vi "Slide Change Display Format.vi"(8 "Error In":errorcluster, 11 "Slide Refnum":refnum<vi>) -> (0 "Error Out":errorcluster)   [LabVIEW 2021, in "GUI.lvlib"]
uses:
  GUI.lvlib
panel:
  # "see the License on the block diagram (Ctrl+E or Window:Show Block Diagram)"
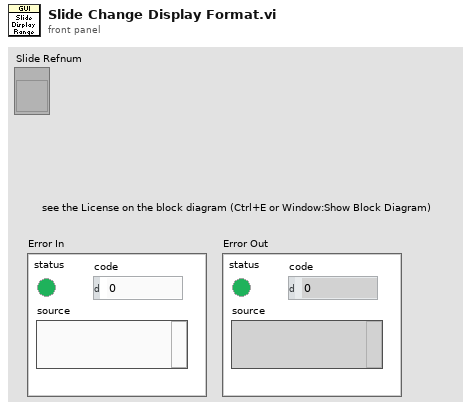
[diagram p1: front panel]
types:
  T1 = typedef "LVFormatAndPrecisionTypeDef.ctl" = cluster{"Format":u8, "Precision":u8}
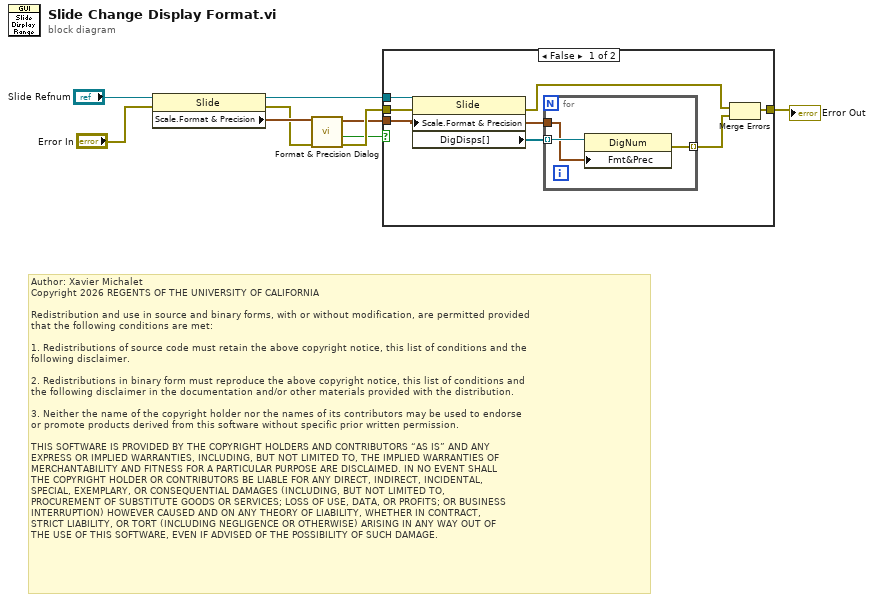
[diagram p0: block diagram]
diagram:
  # "Author: Xavier Michalet\nCopyright 2026 REGENTS OF THE UNIVERSITY OF CALIFORNIA\n\nRedistribution and use in source and binary forms, with or without modification, are permitted provided\nthat the following conditions are met:\n\n1. Redistributions of source code must retain the above copyright notice, this list of conditions and the\nfollowing disclaimer.\n\n2. Redistributions in binary form must reproduce the above copyright notice, this list of conditions and\nthe following disclaimer in the documentation and/or other materials provided with the distribution.\n\n3. Neither the name of the copyright holder nor the names of its contributors may be used to endorse \nor promote products derived from this software without specific prior written permission.\n\nTHIS SOFTWARE IS PROVIDED BY THE COPYRIGHT HOLDERS AND CONTRIBUTORS “AS IS” AND ANY \nEXPRESS OR IMPLIED WARRANTIES, INCLUDING, BUT NOT LIMITED TO, THE IMPLIED WARRANTIES OF\nMERCHANTABILITY AND FITNESS FOR A PARTICULAR PURPOSE ARE DISCLAIMED. IN NO EVENT SHALL\nTHE COPYRIGHT HOLDER OR CONTRIBUTORS BE LIABLE FOR ANY DIRECT, INDIRECT, INCIDENTAL, \nSPECIAL, EXEMPLARY, OR CONSEQUENTIAL DAMAGES (INCLUDING, BUT NOT LIMITED TO, \nPROCUREMENT OF SUBSTITUTE GOODS OR SERVICES; LOSS OF USE, DATA, OR PROFITS; OR BUSINESS\nINTERRUPTION) HOWEVER CAUSED AND ON ANY THEORY OF LIABILITY, WHETHER IN CONTRACT, \nSTRICT LIABILITY, OR TORT (INCLUDING NEGLIGENCE OR OTHERWISE) ARISING IN ANY WAY OUT OF\nTHE USE OF THIS SOFTWARE, EVEN IF ADVISED OF THE POSSIBILITY OF SUCH DAMAGE."
  n1 = property class="Slide"(reference="Slide Refnum", error in="Error In") -> (reference out=w3:refnum<vi>, error out=w6:errorcluster, "Scale.Format & Precision"=w7:T1)
  n2 = call "Format & Precision Dialog.vi"("Error In"=w6, "Display Format in"=w7) -> ("Error Out"=w5:errorcluster, "Cancelled?"=w1:bool, "Display Format out"=w4:T1)  [unwired: 7 in]
  n3 = case shown="False" w1 {
    tunnel: w5 -> [w16 w20]
    tunnel: w4 -> [w13 _]
    tunnel: w3 -> [w15 _]
    tunnel: [w10 w20] -> w2
    frame False {
      n4 = property class="Slide"(reference=w15, error in=w16, "Scale.Format & Precision"=w13) -> (error out=w12:errorcluster, "DigDisps[]"=w14:refnum<vi>[])  [unwired: 1 out]
      n5 = for {
        tunnel: w14 -> [w19] mode=indexing
        tunnel: w13 -> [w18]
        tunnel: [w17] -> w11 mode=indexing
        n6 = property class="DigNum"(reference=w19, "Fmt&Prec"=w18) -> (error out=w17:errorcluster)  [unwired: 1 in, 1 out]
      }
      n7 = Merge Errors(w12, w11) -> (w10:errorcluster)
    }
    frame True {
    }
  }
  "Error Out" <- w2
